vi "HandleRollerPneumatic.vi"(7 "InitState":T1=enum."Middle", 8 "error in (no error)":errorcluster, 11 "Toggle?":bool) -> (0 "error out":errorcluster, 3 "State":T1)   [LabVIEW 2013]
uses:
  DoubleSolenoidAction.ctl
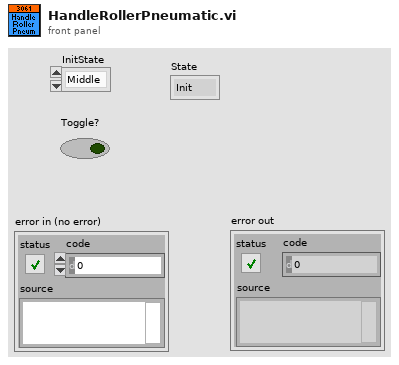
[diagram p1: front panel]
types:
  T1 = typedef "DoubleSolenoidAction.ctl" = enum16{"Init", "Middle", "In", "Out"}
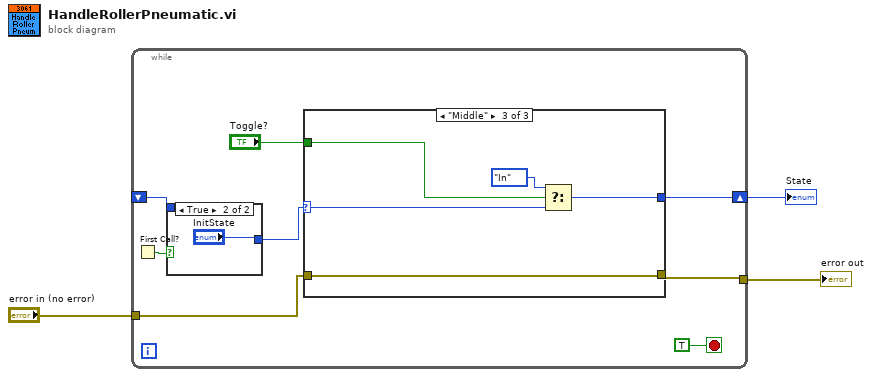
[diagram p0: block diagram]
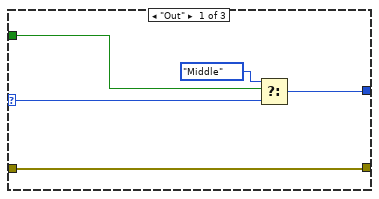
[diagram p3: hidden frame]
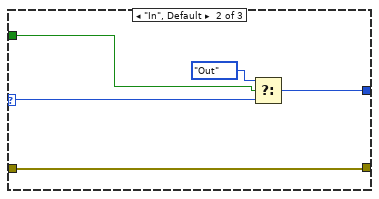
[diagram p4: hidden frame]
diagram:
  n1 = while {
    shift-right: [w10] -> w3
    shift-left: _ -> [w7]
    tunnel: "error in (no error)" -> [w5]
    tunnel: [w4] -> w1
    stop <- TRUE stop-if-true
    n2 = First Call?() -> (First Call?: T/F=w9:bool)
    n3 = case shown="True" w9 {
      tunnel: [w12 "InitState"] -> w8
      tunnel: w7 -> [w12 _]
      frame False {
      }
      frame True {
      }
    }
    n4 = case shown="\"Middle\"" w8 {
      selector: w8 -> [w16 w21 w28]
      tunnel: [w17 w22 w27] -> w10
      tunnel: "Toggle?" -> [w14 w19 w24]
      tunnel: w5 -> [w15 w20 w25]
      tunnel: [w15 w20 w25] -> w4
      frame "Out" {
        n5 = Select(t=DoubleSolenoidAction."Middle", s=w14, f=w16) -> (s? t:f=w17:T1)
      }
      frame "In", Default {
        n6 = Select(t=DoubleSolenoidAction."Out", s=w19, f=w21) -> (s? t:f=w22:T1)
      }
      frame "Middle" {
        n7 = Select(t=DoubleSolenoidAction."In", s=w24, f=w28) -> (s? t:f=w27:T1)
      }
    }
  }
  "State" <- w3
  "error out" <- w1
